vi "MDF4 Create Data Stream.vi"(8 "Error In":errorcluster, 9 "Number of Samples per Read":u32, 10 "Iterations":u32, 11 "Data Group Reference in":i64) -> (0 "Error Out":errorcluster, 1 "Stream Reference out":i64, 3 "Data Group Reference out":i64)   [LabVIEW 2019, in "MD4Logger Engine.lvlib"]
uses:
  MD4Logger Engine.lvlib
  <vilib>/Utility/error.llb/Error Cluster From Error Code.vi
  <vilib>/ErrorRing/Error Ring.xnode
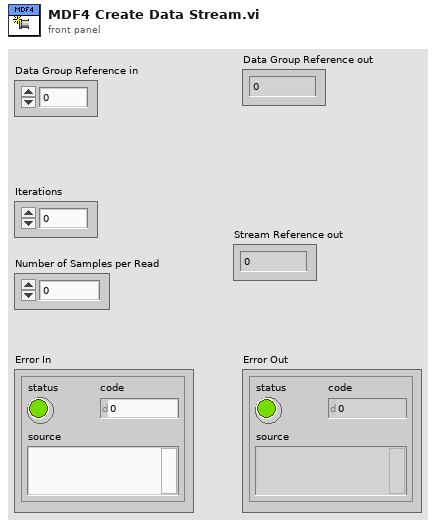
[diagram p1: front panel]
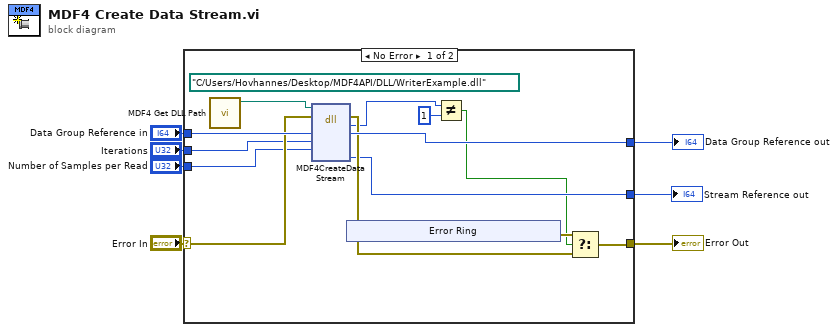
[diagram p0: block diagram]
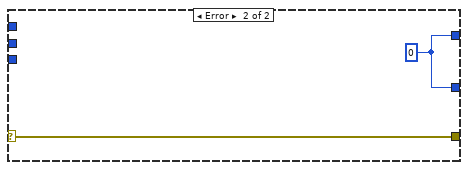
[diagram p2: hidden frame]
diagram:
  n1 = case shown="No Error" "Error In" {
    selector: "Error In" -> [w19 w27]
    tunnel: "Data Group Reference in" -> [w20 _]
    tunnel: [w16 w27] -> w5
    tunnel: [w18 w26] -> w4
    tunnel: "Iterations" -> [w14 _]
    tunnel: [w13 w26] -> w2
    tunnel: "Number of Samples per Read" -> [w12 _]
    frame No Error {
      (unwired) path "C:/Users/Hovhannes/Desktop/MDF4API/DLL/WriterExample.dll" ("path in")
      n2 = call "MDF4 Get DLL Path.vi"() -> ("DLL Path Out"=w8:path)  [unwired: 11 in]
      n3 = dll-call lib="C:/Users/Hovhannes/Desktop/MDF4API/DLL/WriterExample.dll" fn="MDF4CreateDataStream"(path in=w8, error in=w19, "dg"=w20, "iterations"=w14, "num_samples_per_read"=w12) -> (error out=w15:errorcluster, "return type"=w10:i32, "dg"=w18:i64, "DStream"=w13:i64)  [unwired: 4 in, 1 out]
      n4 = xnode "Error Ring"() -> ("error out"=w17:errorcluster)
      n5 = Not Equal?(x=w10, y=1) -> (x != y?=w9:bool)
      n6 = Select(t=w17, s=w9, f=w15) -> (s? t:f=w16:errorcluster)
    }
    frame Error {
      w26 = i64 0 ("m4")
    }
  }
  "Error Out" <- w5
  "Data Group Reference out" <- w4
  "Stream Reference out" <- w2
